vi "Cleanup.vi"(8 "error in (no error)":errorcluster, 11 "ElementEditorPanel in":refnum<class "ElementEditorPanel.lvclass">) -> (0 "error out":errorcluster)   [LabVIEW 2020, in "VolatusGUIEditorCore.lvlib" / "ElementEditorPanel.lvclass"]
uses:
  ElementEditorPanel.lvclass
  ElementEditorPanel.lvclass/ElementEditorPanel.ctl
  lv-oopanel/OOPanel/Panel/Panel.lvclass
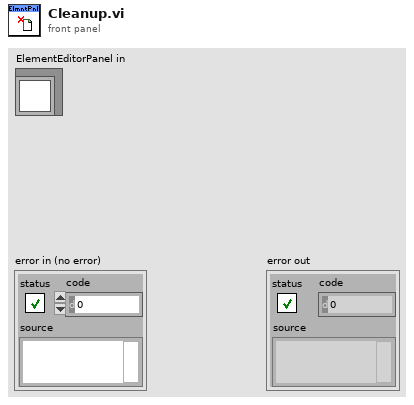
[diagram p1: front panel]
types:
  T1 = typedef "VolatusGUIEditorCore.lvlib/ElementEditorPanel.lvclass/Incoming Events.ctl" = cluster{"Update Control":refnum<user-event>}
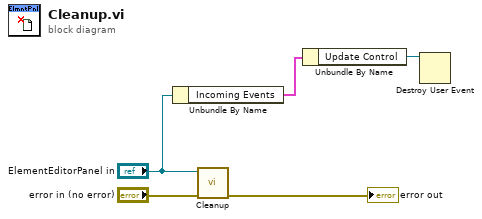
[diagram p0: block diagram]
diagram:
  n1 = Unbundle By Name("ElementEditorPanel in") -> ("Incoming Events"=w2:T1)
  n2 = call-parent "Cleanup.vi"("error in (no error)"="error in (no error)", "Panel in"="ElementEditorPanel in") -> ("error out"=→"error out":errorcluster)  [unwired: 9 in]
  n3 = Unbundle By Name(w2) -> ("Update Control"=w1:refnum<user-event>)
  n4 = Destroy User Event(user event=w1) -> ()  [unwired: 1 in, 1 out]
